vi "Project2_Final_Track_Simulator.vi"() -> ()   [LabVIEW 2016]
uses:
  SubVIs/Global 1.vi
panel:
  in  "Sensor 2 Height\n\n                   in":dbl
  in  "Sensor 1 Height\n\n                   in":dbl
  in  "Simulation Timing":dbl
  out "Total Distance":dbl
  out "Sensor 2 Reading":dbl
  out "Sensor 1 Reading":dbl
  out "Angle":dbl
  out "Elapsed Time":dbl
  out "Y Location":dbl
  out "X Location":dbl
  out "Robot Path":cluster{dbl[], dbl[]}[](graph)
  in  "Robot Width":dbl
  in  "Robot Length":dbl
  in  "Run button":bool
  out "2D Picture":picture
  in  "Sensor 2 Mode":u16(ring) items=["Ambient", "Detect", "Reflected"]
  in  "Sensor 1 Mode":u16(ring) items=["Ambient", "Detect", "Reflected"]
  out "Completed?":bool
  out "Average Speed:":dbl
  in  "Sensor 2 Y Location\n\n                    in":dbl
  in  "Sensor 2 X Location\n\n                    in":dbl
  in  "Sensor 1 Y Location\n\n                    in":dbl
  in  "Sensor 1 X Location\n\n                    in":dbl
  in  "Number of \nColor Sensors":u16(ring) items=["1", "2"]
  in  "Select Track":u16(ring) items=["Final Track", "Final Track, version 2"]
  # "Setup:"
  # "Status:"
  # "Results:"
  # "s"
  # "in"
  # "in"
  # "ft/s"
  # "in"
  # "in"
  # "degrees"
  # "s"
  # "in"
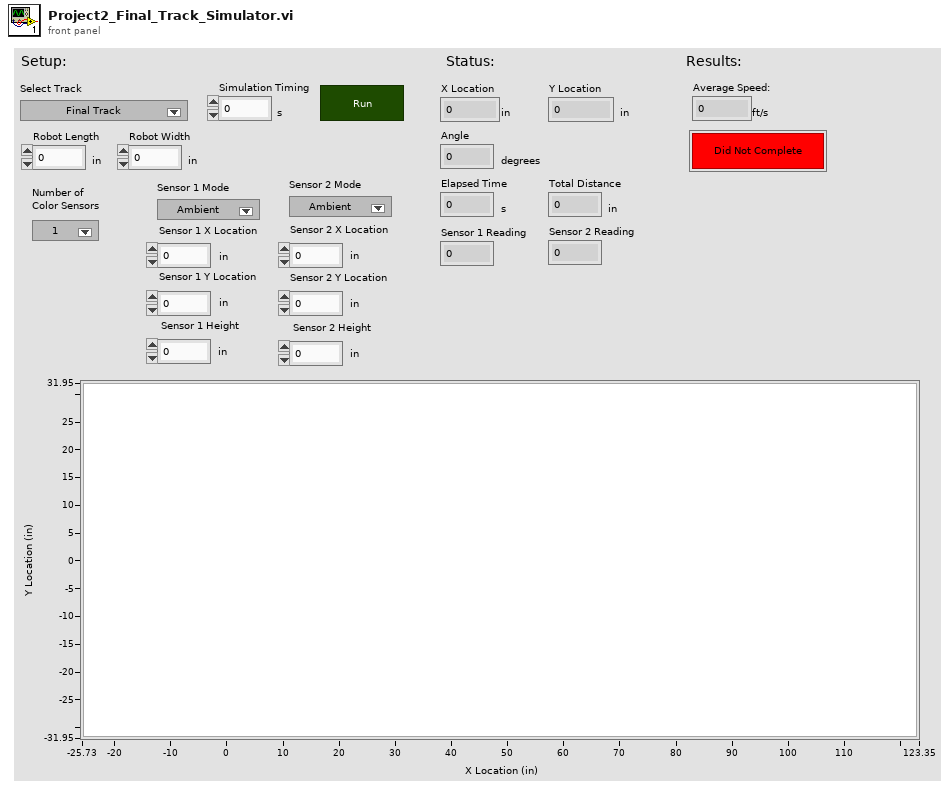
[diagram p1: front panel]
types:
  T1 = typedef "imagedata.ctl" = cluster{"image type":i32, "image depth":i32, "image":u8[], "mask":u8[], "colors":u32[], "Rectangle":cluster{"left":i16, "top":i16, "right":i16, "bottom":i16}}
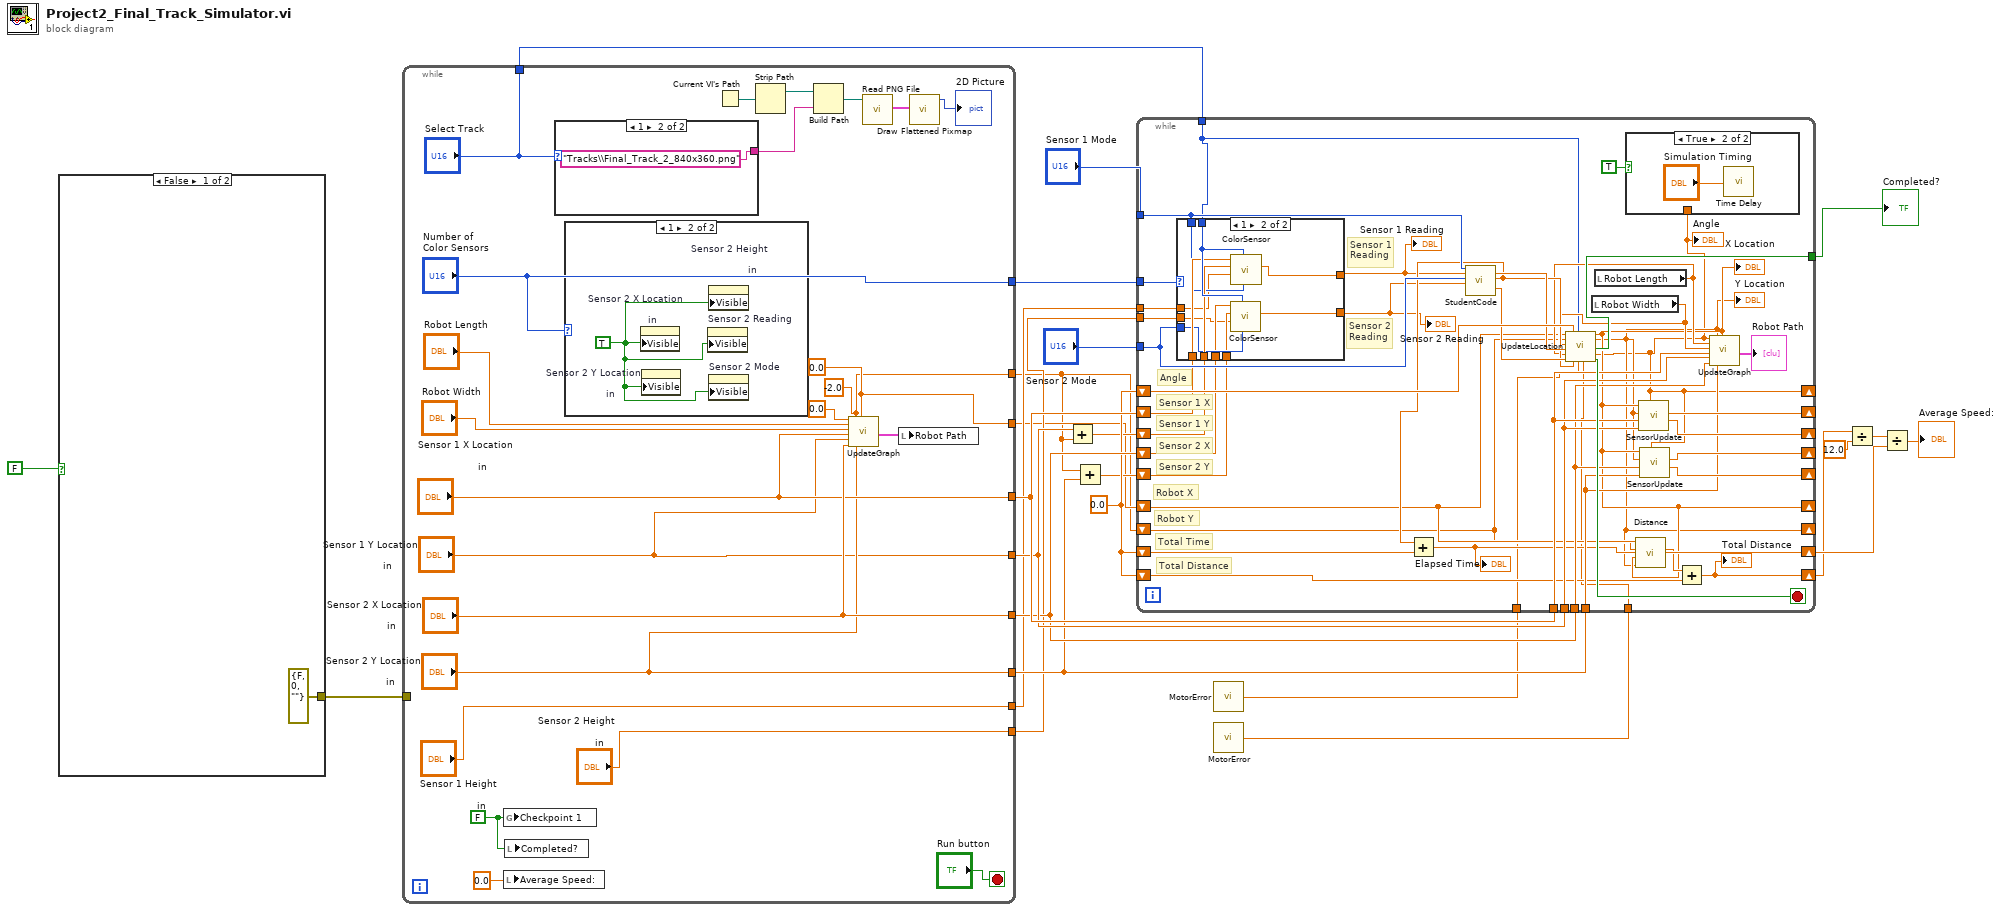
[diagram p0: block diagram]
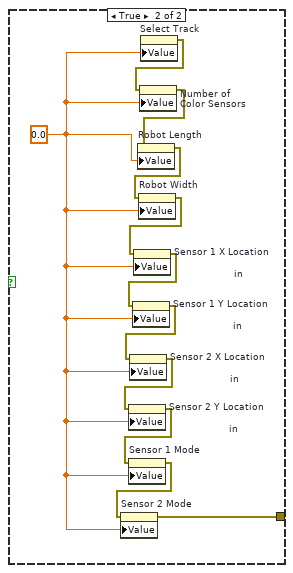
[diagram p2: hidden frame]
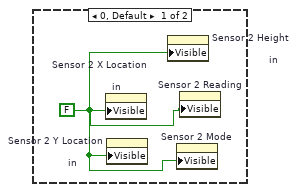
[diagram p3: hidden frame]
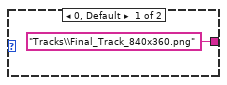
[diagram p4: hidden frame]
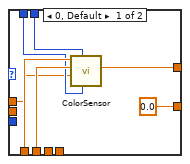
[diagram p6: hidden frame]
diagram:
  w13 = 0.0
  n1 = case shown="False" FALSE {
    tunnel: [errorcluster {"status"=FALSE, "code"=0, "source"=""} ("error out") w27] -> w14
    frame False {
    }
    frame True {
      w37 = 0.0
      n2 = property on="Select Track" class="Ring (strict)"("Value"=w37) -> (error out=w36:errorcluster)  [unwired: 2 in, 1 out]
      n3 = property on="Number of \nColor Sensors" class="Ring (strict)"(error in=w36, "Value"=w37) -> (error out=w35:errorcluster)  [unwired: 1 in, 1 out]
      n4 = property on="Robot Length" class="DigNum (strict)"(error in=w35, "Value"=w37) -> (error out=w34:errorcluster)  [unwired: 1 in, 1 out]
      n5 = property on="Robot Width" class="DigNum (strict)"(error in=w34, "Value"=w37) -> (error out=w33:errorcluster)  [unwired: 1 in, 1 out]
      n6 = property on="Sensor 1 X Location\n\n                    in" class="DigNum (strict)"(error in=w33, "Value"=w37) -> (error out=w32:errorcluster)  [unwired: 1 in, 1 out]
      n7 = property on="Sensor 1 Y Location\n\n                    in" class="DigNum (strict)"(error in=w32, "Value"=w37) -> (error out=w31:errorcluster)  [unwired: 1 in, 1 out]
      n8 = property on="Sensor 2 X Location\n\n                    in" class="DigNum (strict)"(error in=w31, "Value"=w37) -> (error out=w30:errorcluster)  [unwired: 1 in, 1 out]
      n9 = property on="Sensor 2 Y Location\n\n                    in" class="DigNum (strict)"(error in=w30, "Value"=w37) -> (error out=w29:errorcluster)  [unwired: 1 in, 1 out]
      n10 = property on="Sensor 1 Mode" class="Ring (strict)"(error in=w29, "Value"=w37) -> (error out=w28:errorcluster)  [unwired: 1 in, 1 out]
      n11 = property on="Sensor 2 Mode" class="Ring (strict)"(error in=w28, "Value"=w37) -> (error out=w27:errorcluster)  [unwired: 1 in, 1 out]
    }
  }
  n12 = while {
    tunnel: ["Number of \nColor Sensors"] -> w25
    tunnel: ["Select Track"] -> w24
    tunnel: ["Sensor 1 X Location\n\n                    in"] -> w21
    tunnel: ["Sensor 1 Y Location\n\n                    in"] -> w20
    tunnel: ["Sensor 2 X Location\n\n                    in"] -> w19
    tunnel: ["Sensor 2 Y Location\n\n                    in"] -> w18
    tunnel: w14 -> [_]
    tunnel: [w42] -> w1
    tunnel: ["Sensor 1 Height\n\n                   in"] -> w6
    tunnel: ["Sensor 2 Height\n\n                   in"] -> w5
    tunnel: [w44] -> w2
    stop <- "Run button" stop-if-true
    w39 = FALSE
    w44 = 0.0 ("Angle")
    w42 = -2.0 ("Angle")
    n13 = global write "Global 1.vi" "Checkpoint 1"(w39) -> ()
    n14 = local write "Average Speed:"(0.0 ("Average Speed:")) -> ()
    n15 = local write "Completed?"(w39) -> ()
    n16 = case shown="1" "Select Track" {
      tunnel: ["Tracks\\Final_Track_840x360.png" "Tracks\\Final_Track_2_840x360.png"] -> w57
      frame 0, Default {
      }
      frame 1 {
      }
    }
    n17 = case shown="1" "Number of \nColor Sensors" {
      frame 0, Default {
        w61 = FALSE ("Visible")
        n18 = property on="Sensor 2 X Location\n\n                    in" class="DigNum (strict)"("Visible"=w61) -> ()  [unwired: 2 in, 2 out]
        n19 = property on="Sensor 2 Y Location\n\n                    in" class="DigNum (strict)"("Visible"=w61) -> ()  [unwired: 2 in, 2 out]
        n20 = property on="Sensor 2 Height\n\n                   in" class="DigNum (strict)"("Visible"=w61) -> ()  [unwired: 2 in, 2 out]
        n21 = property on="Sensor 2 Mode" class="Ring (strict)"("Visible"=w61) -> ()  [unwired: 2 in, 2 out]
        n22 = property on="Sensor 2 Reading" class="DigNum (strict)"("Visible"=w61) -> ()  [unwired: 2 in, 2 out]
      }
      frame 1 {
        w62 = TRUE ("Visible")
        n23 = property on="Sensor 2 X Location\n\n                    in" class="DigNum (strict)"("Visible"=w62) -> ()  [unwired: 2 in, 2 out]
        n24 = property on="Sensor 2 Y Location\n\n                    in" class="DigNum (strict)"("Visible"=w62) -> ()  [unwired: 2 in, 2 out]
        n25 = property on="Sensor 2 Reading" class="DigNum (strict)"("Visible"=w62) -> ()  [unwired: 2 in, 2 out]
        n26 = property on="Sensor 2 Height\n\n                   in" class="DigNum (strict)"("Visible"=w62) -> ()  [unwired: 2 in, 2 out]
        n27 = property on="Sensor 2 Mode" class="Ring (strict)"("Visible"=w62) -> ()  [unwired: 2 in, 2 out]
      }
    }
    n28 = Current VI's Path() -> (path=w58:path)
    n29 = Strip Path(path=w58) -> (stripped path=w47:path)  [unwired: 1 out]
    n30 = Build Path(base path=w47, name or relative path=w57) -> (appended path=w56:path)
    n31 = call "UpdateGraph.vi"("Angle"=0.0, "Robot Length"="Robot Length", "Robot Width"="Robot Width", "Sensor 1 X"="Sensor 1 X Location\n\n                    in", "Sensor 1 Y"="Sensor 1 Y Location\n\n                    in", "Sensor 2 X"="Sensor 2 X Location\n\n                    in", "Robot Y"=w42, "Sensor 2 Y"="Sensor 2 Y Location\n\n                    in", "Robot X"=w44) -> ("appended array"=w59:cluster{dbl[], dbl[]}[])  [unwired: 10 in]
    n32 = call <vilib>:"Read PNG File.vi"("path to PNG file"=w56) -> ("image data"=w55:T1)  [unwired: 8 in, 2 out]
    n33 = local write "Robot Path"(w59) -> ()
    n34 = call <vilib>:"Draw Flattened Pixmap.vi"("image data"=w55) -> ("new picture"=→"2D Picture":picture)  [unwired: 8 in]
  }
  n35 = Add(x=w20, y=w1) -> (x+y=w4:dbl)
  n36 = Add(x=w1, y=w18) -> (x+y=w3:dbl)
  n37 = call "MotorError.vi"() -> ("Motor Error Value"=w8:dbl)
  n38 = call "MotorError.vi"() -> ("Motor Error Value"=w7:dbl)
  n39 = while {
    shift-right: [w76] -> _
    shift-left: w2 -> [w78]
    shift-right: [w71] -> _
    shift-left: w1 -> [w77]
    tunnel: w25 -> [w105]
    tunnel: w24 -> [w82]
    shift-right: [w102] -> _
    shift-left: w21 -> [w75]
    shift-right: [w101] -> _
    shift-left: w4 -> [w74]
    shift-right: [w100] -> _
    shift-left: w19 -> [w73]
    shift-right: [w99] -> _
    shift-left: w3 -> [w72]
    shift-right: [w65] -> _
    shift-left: w13 -> [w104]
    tunnel: "Sensor 1 Mode" -> [w94]
    tunnel: "Sensor 2 Mode" -> [w93]
    tunnel: w21 -> [w98]
    tunnel: w20 -> [w97]
    tunnel: w19 -> [w96]
    tunnel: w18 -> [w95]
    tunnel: [w90] -> w17
    shift-right: [w85] -> w15
    shift-left: w13 -> [w89]
    shift-right: [w79] -> w12
    shift-left: w13 -> [w81]
    tunnel: w8 -> [w70]
    tunnel: w7 -> [w69]
    tunnel: w6 -> [w68]
    tunnel: w5 -> [w67]
    stop <- w103 stop-if-true
    # "Total Distance"
    # "Total Time"
    # "Sensor 2\nReading"
    # "Sensor 1\nReading"
    # "Sensor 2 Y"
    # "Sensor 2 X"
    # "Sensor 1 Y"
    # "Sensor 1 X"
    # "Angle"
    # "Robot Y"
    # "Robot X"
    n40 = case shown="1" w105 {
      tunnel: [w114 w125] -> w84
      tunnel: [0.0 ("Color Sensor Reading") w124] -> w83
      tunnel: w82 -> [w112 w123]
      tunnel: w75 -> [w111 w121]
      tunnel: w74 -> [w110 w122]
      tunnel: w94 -> [w109 w120]
      tunnel: w93 -> [_ w119]
      tunnel: w73 -> [_ w118]
      tunnel: w72 -> [_ w117]
      tunnel: w68 -> [w108 w116]
      tunnel: w67 -> [_ w115]
      frame 0, Default {
        n41 = call "ColorSensor.vi"("Sensor Mode"=w109, "Select Track"=w112, "Height"=w108, "Y Location Sensor"=w110, "X Location Sensor"=w111) -> ("Color Sensor Reading"=w114:dbl)  [unwired: 6 in]
      }
      frame 1 {
        n42 = call "ColorSensor.vi"("Sensor Mode"=w119, "Select Track"=w123, "Height"=w115, "Y Location Sensor"=w117, "X Location Sensor"=w118) -> ("Color Sensor Reading"=w124:dbl)  [unwired: 6 in]
        n43 = call "ColorSensor.vi"("Sensor Mode"=w120, "Select Track"=w123, "Height"=w116, "Y Location Sensor"=w122, "X Location Sensor"=w121) -> ("Color Sensor Reading"=w125:dbl)  [unwired: 6 in]
      }
    }
    "Sensor 1 Reading" <- w84
    "Sensor 2 Reading" <- w83
    n44 = call "StudentCode.vi"("Sensor 1 Mode"=w94, "Sensor 1 Value"=w84, "Sensor 2 Mode"=w93, "Sensor 2 Value"=w83) -> ("Motor 1 Value"=w92:dbl, "Motor On Duration"=w88:dbl, "Motor 2 Value"=w91:dbl)  [unwired: 13 in]
    n45 = Add(x=w88, y=w89) -> (x+y=w85:dbl)
    "Elapsed Time" <- w85
    n46 = local read "Robot Width"() -> (w87:dbl)
    n47 = local read "Robot Length"() -> (w86:dbl)
    n48 = call "UpdateLocation.vi"("Robot X Location"=w78, "Robot Y Location"=w77, "Robot Width"=w87, "Motor 1 Value"=w92, "Robot Length"=w86, "Motor 2 Value"=w91, "Angle"=w104, "Motor On Duration"=w88, "Select Track"=w82, "Motor 1 Error"=w70, "Motor 2 Error"=w69) -> ("New Robot X Location"=w76:dbl, "New Robot Y Location"=w71:dbl, "Complete?"=w90:bool, "New Angle"=w65:dbl, "Terminate?"=w103:bool)  [unwired: 4 in]
    "X Location" <- w76
    "Y Location" <- w71
    "Angle" <- w65
    n49 = case shown="True" TRUE {
      tunnel: w65 -> [_ _]
      frame False {
      }
      frame True {
        n50 = call "Time Delay"("Delay Time (s)"="Simulation Timing") -> ()  [unwired: 10 in, 1 out]
      }
    }
    n51 = call "Distance.vi"("New y"=w71, "New X"=w76, "Original y"=w77, "Original X"=w78) -> ("Distance"=w80:dbl)  [unwired: 7 in]
    n52 = call "SensorUpdate.vi"("Angle"=w65, "Sensor Y"=w97, "Sensor X"=w98, "Robot Y"=w71, "Robot X"=w76) -> ("New Sensor Y"=w101:dbl, "New Sensor X"=w102:dbl)  [unwired: 5 in]
    n53 = call "SensorUpdate.vi"("Angle"=w65, "Sensor Y"=w95, "Sensor X"=w96, "Robot Y"=w71, "Robot X"=w76) -> ("New Sensor Y"=w99:dbl, "New Sensor X"=w100:dbl)  [unwired: 5 in]
    n54 = Add(x=w80, y=w81) -> (x+y=w79:dbl)
    "Total Distance" <- w79
    n55 = call "UpdateGraph.vi"("Angle"=w65, "Robot Length"=w86, "Robot Width"=w87, "Sensor 1 X"=w98, "Sensor 1 Y"=w97, "Sensor 2 X"=w96, "Robot Y"=w71, "Sensor 2 Y"=w95, "Robot X"=w76) -> ("appended array"=→"Robot Path":cluster{dbl[], dbl[]}[])  [unwired: 10 in]
  }
  "Completed?" <- w17
  n56 = Divide(x=w12, y=12.0) -> (x/y=w11:dbl)
  n57 = Divide(x=w11, y=w15) -> (x/y=→"Average Speed:":dbl)
